vi "XML Script - StaticVIReference.vi"(0 "x":i32=-1, 1 "y":i32=-1, 2 "out":i32=-1, 4 "path":path, 6 "name":string, 8 "Static VI Reference Type":T1, 9 "prefix (name)":string, 10 "in":i32=-1) -> (5 "name (wire source)":string, 7 "XML Script Command - Function":string)   [LabVIEW 2017]
uses:
  <vilib>/_script/XML Scripting/XML Script - StaticVIReferenceType.ctl
  <vilib>/_script/XML Scripting/XML Script Attribute.ctl
  <vilib>/_script/XML Scripting/XML Script Tag.ctl
  <vilib>/_script/XML Scripting/XML Script - PathToXMLString.vi
panel:
  # "position"
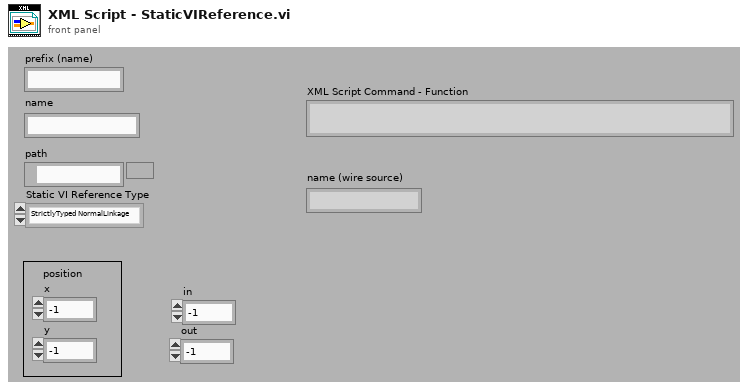
[diagram p1: front panel]
types:
  T1 = typedef "XML Script - StaticVIReferenceType.ctl" = enum16{"StrictlyTyped NormalLinkage", "NonStrictlyTyped NormalLinkage", "StrictlyTyped WeakLinkage", "NonStrictlyTyped WeakLinkage"}
  T2 = typedef "XML Script Attribute.ctl" = enum16{"name", "style", "path", "position", "in", "out", "width", "height", "index", "value", "default", "location", "offset", "typeindex", "size", "source", "destination", "indicator", "type", "controlname", "label", "conpaneidx", "mode", "description", "hasCondTerm", "linkIdentity", "caseselectortype", "concatInputs", "inName", "instantiationpath", "loopCondition", "IndexMode", "formulaInputs", "formulaOutputs", "msnFuncName", "msnIsDynamic", "msnIsODEUserFunction", "ignoreSearchDialog"}
  T3 = typedef "XML Script Tag.ctl" = enum16{"Script", "Function", "SubVI", "GrowableFunction", "Structure", "MultiframeStructure", "Frame", "Tunnel", "ShiftRegister", "Constant", "Control", "Terminal", "Wire", "StaticVIReference", "ControlTerminal", "CompoundArithmetic", "FlatSequence", "FlatSequenceFrame", "MathScriptCallByRef", "BuildArray", "GenericSubVI", "MathScriptNode"}
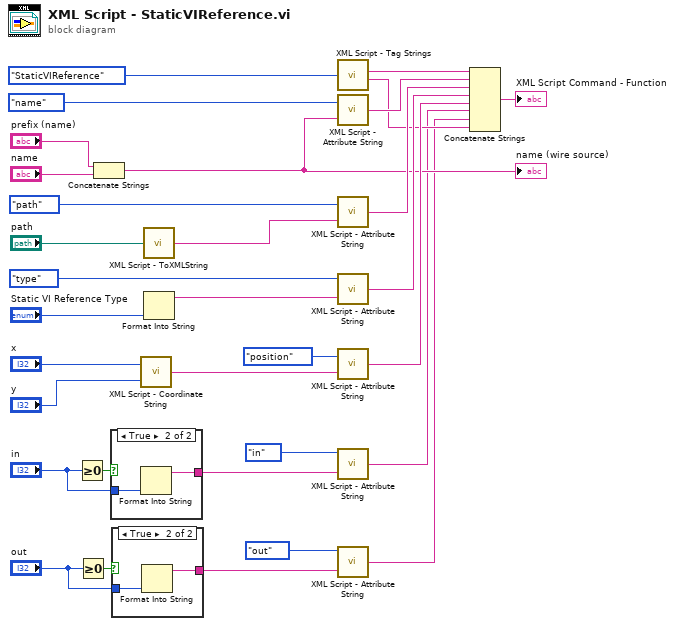
[diagram p0: block diagram]
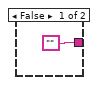
[diagram p2: hidden frame]
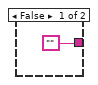
[diagram p3: hidden frame]
diagram:
  n1 = Greater Or Equal To 0?(x="in") -> (x >= 0?=w7:bool)
  n2 = Greater Or Equal To 0?(x="out") -> (x >= 0?=w11:bool)
  n3 = Concatenate Strings("prefix (name)", "name") -> (w16:string)
  "name (wire source)" <- w16
  n4 = case shown="True" w7 {
    tunnel: "in" -> [_ w35]
    tunnel: ["" w34] -> w9
    frame False {
    }
    frame True {
      n5 = Format Into String(w35) -> (resulting string=w34:string)  [unwired: 3 in, 1 out]
    }
  }
  n6 = case shown="True" w11 {
    tunnel: "out" -> [_ w38]
    tunnel: ["" w37] -> w13
    frame False {
    }
    frame True {
      n7 = Format Into String(w38) -> (resulting string=w37:string)  [unwired: 3 in, 1 out]
    }
  }
  n8 = call <vilib>:"XML Script - Coordinate String.vi"("y"="y", "x"="x") -> ("(x,y)"=w29:string)
  n9 = call-poly <vilib>:"XML Script - ToXMLString.vi"("Path"="path") -> ("Valid XML String (out)"=w2:string)
  n10 = Format Into String("Static VI Reference Type") -> (resulting string=w14:string)  [unwired: 3 in, 1 out]
  n11 = call <vilib>:"XML Script - Tag Strings.vi"("XML Script Tag"=XML_Script_Tag."StaticVIReference") -> ("XML String - Begin Tag"=w26:string, "XML String - End Tag"=w5:string)  [unwired: 2 in]
  n12 = call <vilib>:"XML Script - Attribute String.vi"("Attribute String"=w16, "XML Script Attribute"=XML_Script_Attribute."name") -> ("XML Script - Attribute String"=w24:string)
  n13 = call <vilib>:"XML Script - Attribute String.vi"("Attribute String"=w2, "XML Script Attribute"=XML_Script_Attribute."path") -> ("XML Script - Attribute String"=w22:string)
  n14 = call <vilib>:"XML Script - Attribute String.vi"("Attribute String"=w14, "XML Script Attribute"=XML_Script_Attribute."type") -> ("XML Script - Attribute String"=w19:string)
  n15 = call <vilib>:"XML Script - Attribute String.vi"("Attribute String"=w29, "XML Script Attribute"=XML_Script_Attribute."position") -> ("XML Script - Attribute String"=w21:string)
  n16 = call <vilib>:"XML Script - Attribute String.vi"("Attribute String"=w9, "XML Script Attribute"=XML_Script_Attribute."in") -> ("XML Script - Attribute String"=w4:string)
  n17 = call <vilib>:"XML Script - Attribute String.vi"("Attribute String"=w13, "XML Script Attribute"=XML_Script_Attribute."out") -> ("XML Script - Attribute String"=w3:string)
  n18 = Concatenate Strings(w26, w24, w22, w19, w21, w4, w3, w5) -> (→"XML Script Command - Function":string)
